vi "LEP_RV_CGen.vi"(7 "Rebuild":bool, 8 "error in (no error)":errorcluster, 9 "Top Level VI":path, 10 "Destination Folder":path, 11 "Configuration":T2={"Enable debugging"=FALSE, "Debug Options"=0, "Use stack variables"=FALSE, "Generate serial only"=FALSE, "Generate guard code"=TRUE, "Generate Integer Only"=TRUE, "Generate C Function Calls"=TRUE, "ExpressionFolding"=FALSE, "Constant Allocation"=0, "Constant Deallocation"=0, "Build Specification ID"="", "Preprocessor symbols (define)"="", "Compiler Flags"="", "Linker Flags"="", "Mode"=1, "Optimization"=2, "Optimize for time"=FALSE, "Enable cross-module optimization"=FALSE, "Include paths"=[], "Optimize heap size"=TRUE, "Use MicroLib"=FALSE, "Debug Mode"=2, "Enable profile information"=FALSE, "Host name"="board", "Use DHCP"=TRUE, "IP address"="0.0.0.0", "Subnet mask"="", "Gateway"="0.0.0.0", "Primary DNS"="0.0.0.0", "Secondary DNS"="0.0.0.0", "MAC in target memory"=TRUE, "MAC address"="", "Console output"=1, "Target serial port"=1} {"Constant Deallocation" items=["Out of Scope", "VI End", "Application End"]; "Constant Allocation" items=["First Use", "Containing Loop", "VI Initialization", "Application Initialization"]; "Target serial port" items=["0", "1", "2", "3"]; "Console output" items=["Processor status window", "Serial port"]; "Optimization" items=["Level 0 (-O0)", "Level 1 (-O1)", "Level 2 (-O2)", "Level 3 (-O3)"]; "Mode" items=["ARM-Mode", "Thumb-Mode"]; "Debug Options" items=["Use ULINK Debugger", "Use Simulator"]; "Debug Mode" items=["Instrumented (serial port)", "Instrumented (TCP/IP)", "Non-instrumented (JTAG/USB)"]}) -> (0 "error out":errorcluster, 1 "Error Indicator":bool[](array[boolean]), 2 "Status":T3(ring)=enum."EmptyTopLevelVIPath", 3 "Configuration":T2={"Enable debugging"=FALSE, "Debug Options"=0, "Use stack variables"=FALSE, "Generate serial only"=FALSE, "Generate guard code"=TRUE, "Generate Integer Only"=TRUE, "Generate C Function Calls"=TRUE, "ExpressionFolding"=FALSE, "Constant Allocation"=0, "Constant Deallocation"=0, "Build Specification ID"="", "Preprocessor symbols (define)"="", "Compiler Flags"="", "Linker Flags"="", "Mode"=1, "Optimization"=2, "Optimize for time"=FALSE, "Enable cross-module optimization"=FALSE, "Include paths"=[], "Optimize heap size"=TRUE, "Use MicroLib"=FALSE, "Debug Mode"=2, "Enable profile information"=FALSE, "Host name"="board", "Use DHCP"=TRUE, "IP address"="0.0.0.0", "Subnet mask"="", "Gateway"="0.0.0.0", "Primary DNS"="0.0.0.0", "Secondary DNS"="0.0.0.0", "MAC in target memory"=TRUE, "MAC address"="", "Console output"=1, "Target serial port"=1} {"Constant Deallocation" items=["Out of Scope", "VI End", "Application End"]; "Constant Allocation" items=["First Use", "Containing Loop", "VI Initialization", "Application Initialization"]; "Target serial port" items=["0", "1", "2", "3"]; "Console output" items=["Processor status window", "Serial port"]; "Optimization" items=["Level 0 (-O0)", "Level 1 (-O1)", "Level 2 (-O2)", "Level 3 (-O3)"]; "Mode" items=["ARM-Mode", "Thumb-Mode"]; "Debug Options" items=["Use ULINK Debugger", "Use Simulator"]; "Debug Mode" items=["Instrumented (serial port)", "Instrumented (TCP/IP)", "Non-instrumented (JTAG/USB)"]}, 4 "Node ID List":i32[](array[numeric]), 5 "Message List":string[][](array[string]))   [LabVIEW 2011]
doc: "Invokes the LabVIEW C Code Generator. This VI is a wrapper VI for the GenerateCCodeVariant VI server call."
uses:
  LEP_RV_Config.ctl
  LEP_RV_CGen.ctl
  <vilib>/LabVIEW Targets/Embedded/Debug/DD/utils/EMB_Debug_DD_GetSetAttrib_Numeric.vi
panel:
  in  "Config":T1={"TargetName"="", "GenerateDebugInfo"=FALSE, "GenerateGuardCode"=FALSE, "GenerateSerialOnly"=FALSE, "UseStackVariables"=FALSE, "MemoryModel"=0, "DestinationFolder"=path "", "GenerateIntegerOnly"=FALSE, "interruptServiceRoutineVIs"=[], "GenerateInlinePrintf"=FALSE, "BigEndian"=FALSE, "GenerateCFunctionCalls"=FALSE, "IncrementalBuild"=FALSE, "OCDIComments"=FALSE, "TargetAlignment"=8, "dynamicVIs"=[], "ExpressionFolding"=FALSE, "ProfileEnable"=FALSE, "Optimize subVI calls"=FALSE, "ConstantAllocation"=0, "ConstantDeallocation"=0, "VariableManagerIP"="", "BuildSpecID"="", "Silent"=TRUE} {"ConstantDeallocation" items=["Out of Scope", "VI End", "Application End"]; "ConstantAllocation" items=["First Use", "Containing Loop", "VI Initialization", "Application Initialization"]}
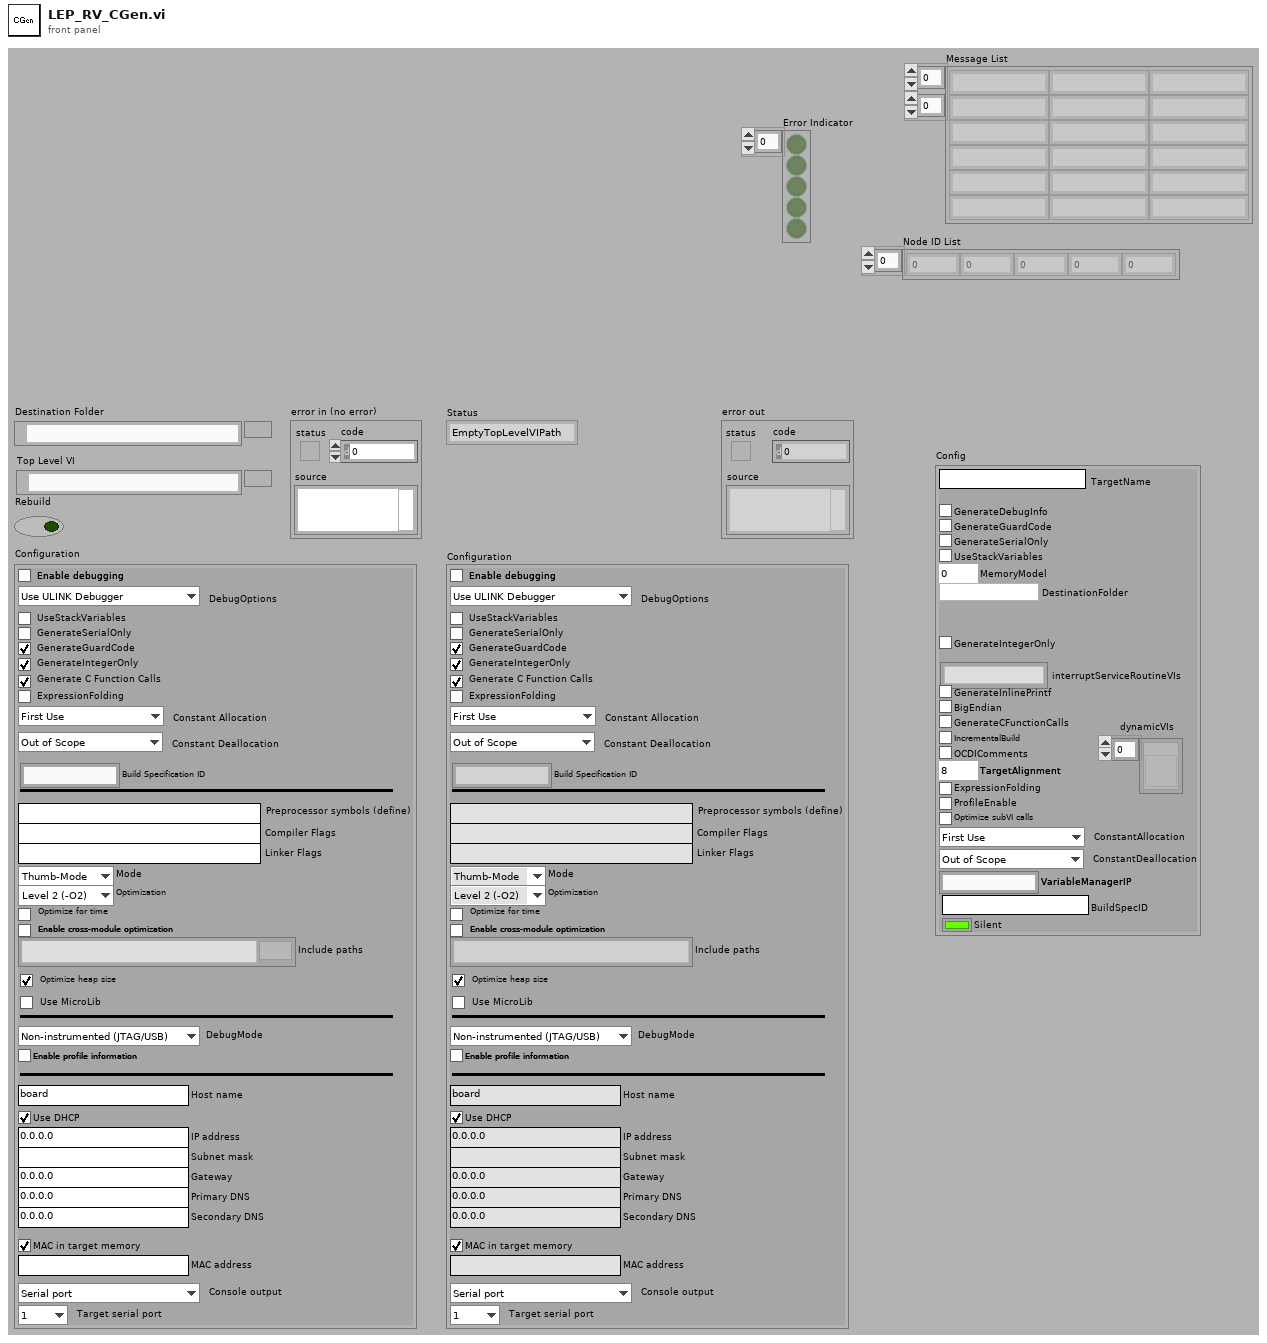
[diagram p1: front panel]
types:
  T1 = typedef "LEP_RV_CGen.ctl" = cluster{"TargetName":string, "GenerateDebugInfo":bool, "GenerateGuardCode":bool, "GenerateSerialOnly":bool, "UseStackVariables":bool, "MemoryModel":i32, "DestinationFolder":path, "GenerateIntegerOnly":bool, "interruptServiceRoutineVIs":path[], "GenerateInlinePrintf":bool, "BigEndian":bool, "GenerateCFunctionCalls":bool, "IncrementalBuild":bool, "OCDIComments":bool, "TargetAlignment":i32, "dynamicVIs":refnum<vi>[], "ExpressionFolding":bool, "ProfileEnable":bool, "Optimize subVI calls":bool, "ConstantAllocation":u16, "ConstantDeallocation":u16, "VariableManagerIP":string, "BuildSpecID":string, "Silent":bool}
  T2 = typedef "LEP_RV_Config.ctl" = cluster{"Enable debugging":bool, "Debug Options":u16, "Use stack variables":bool, "Generate serial only":bool, "Generate guard code":bool, "Generate Integer Only":bool, "Generate C Function Calls":bool, "ExpressionFolding":bool, "Constant Allocation":u16, "Constant Deallocation":u16, "Build Specification ID":string, "Preprocessor symbols (define)":string, "Compiler Flags":string, "Linker Flags":string, "Mode":u16, "Optimization":u16, "Optimize for time":bool, "Enable cross-module optimization":bool, "Include paths":path[], "Optimize heap size":bool, "Use MicroLib":bool, "Debug Mode":u16, "Enable profile information":bool, "Host name":string, "Use DHCP":bool, "IP address":string, "Subnet mask":string, "Gateway":string, "Primary DNS":string, "Secondary DNS":string, "MAC in target memory":bool, "MAC address":string, "Console output":u16, "Target serial port":u16}
  T3 = enum16{"NoErr", "TopLevelVIErr", "EmptyTopLevelVIPath", "CGenErr", "CpySuppFilesErr", "ProjectInfoErr", "NoTopLevelVIErr", "CreateBuildFolderErr", "EmptyBuildFolderErr", "LoadConfigErr", "BildToolsErr", "CompileErr", "LinkError", "DebugInfoErr", "NotFoundErr", "AccessErr", "ExecErr", "UnknownErr", "ISRErr"}
  T4 = enum16{"NoErr", "TopLevelVIErr", "EmptyTopLevelVIPath", "CGenErr", "CpySuppFilesErr", "ProjectInfoErr", "NoTopLevelVIErr", "CreateBuildFolderErr", "EmptyBuildFolderErr", "LoadConfigErr", "BildToolsErr", "CompileErr", "LinkError", "DebugInfoErr", "NotFoundErr", "AccessErr", "ExecErr", "UnknownErr"}
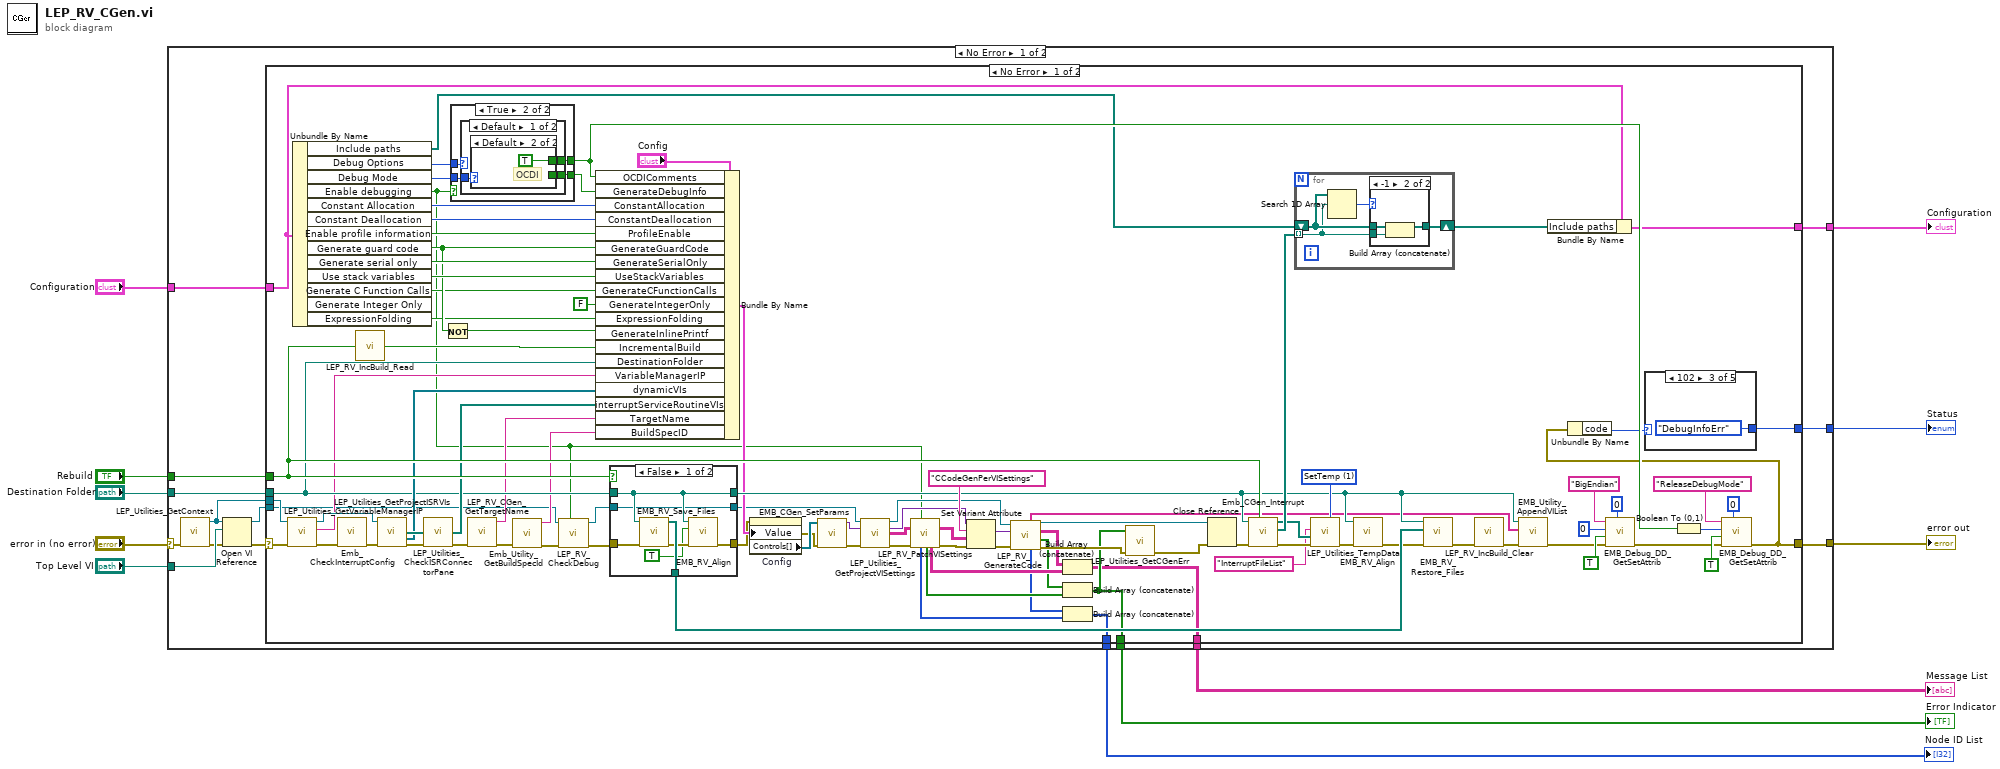
[diagram p0: block diagram]
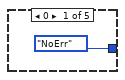
[diagram p2: hidden frame]
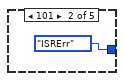
[diagram p3: hidden frame]
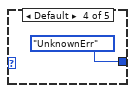
[diagram p4: hidden frame]
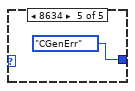
[diagram p5: hidden frame]
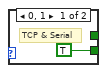
[diagram p7: hidden frame]
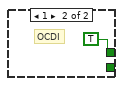
[diagram p8: hidden frame]
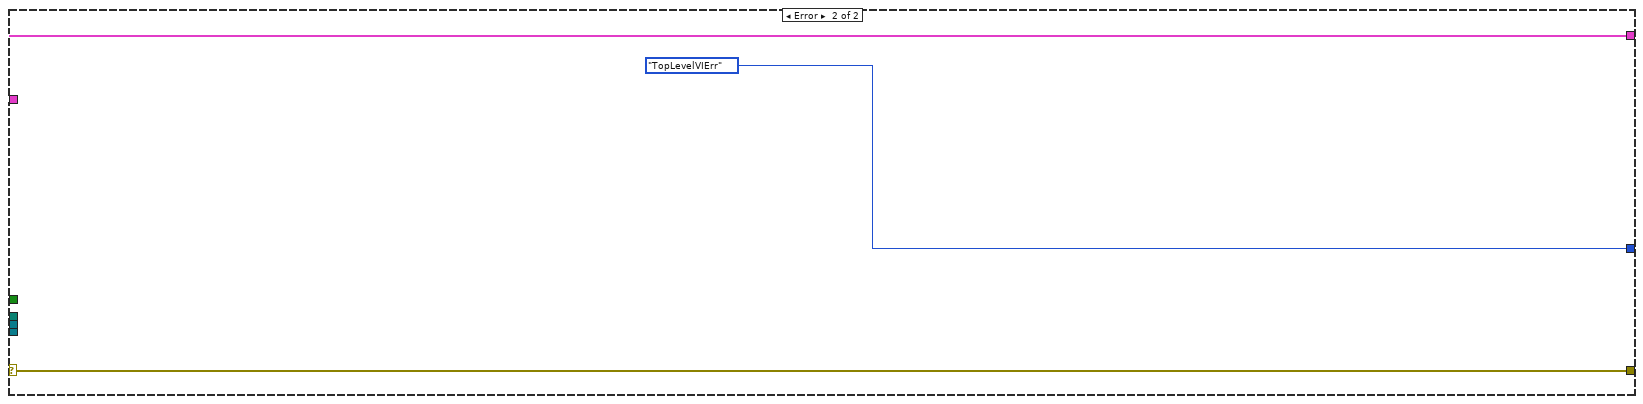
[diagram p11: hidden frame]
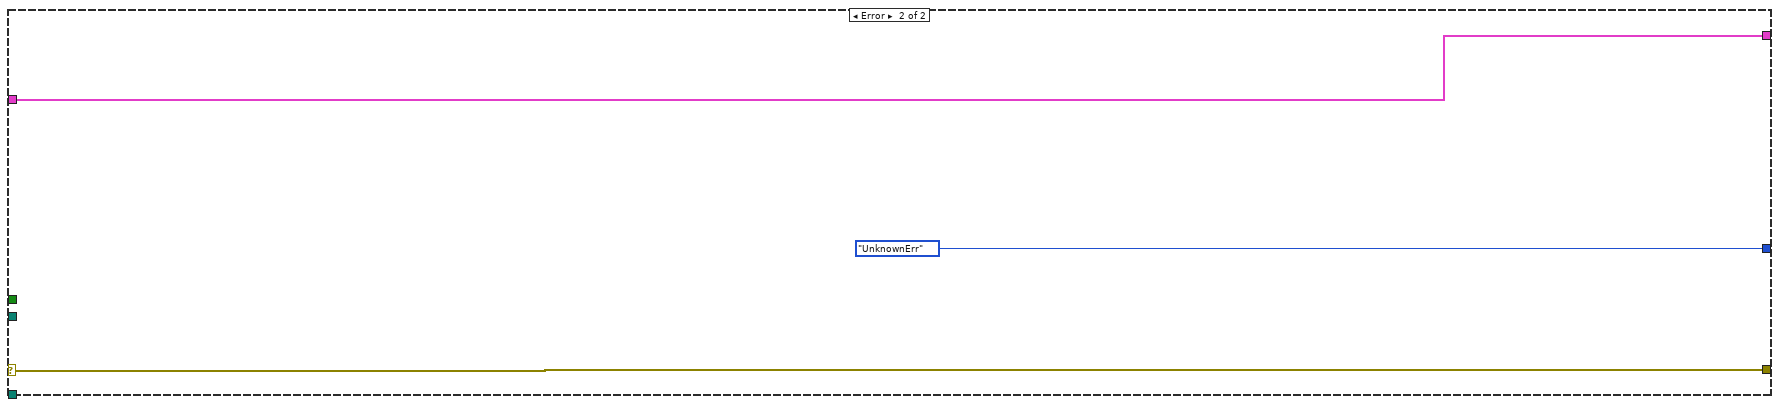
[diagram p12: hidden frame]
diagram:
  n1 = case shown="No Error" "error in (no error)" {
    selector: "error in (no error)" -> [w14 w160]
    tunnel: [w13 w160] -> w7
    tunnel: "Top Level VI" -> [w26 _]
    tunnel: "Destination Folder" -> [w24 _]
    tunnel: "Configuration" -> [w15 w158]
    tunnel: [w22 T4."UnknownErr" ("Errors")] -> w6
    tunnel: [w21 w158] -> w5
    tunnel: "Rebuild" -> [w19 _]
    tunnel: [w18 _] -> w1
    tunnel: [w17 _] -> w3
    tunnel: [w16 _] -> w2
    frame No Error {
      n2 = call <vilib>:"LEP_Utilities_GetContext.vi"("error in"=w14) -> ("error out"=w12:errorcluster, "Context"=w20:refnum<vi>)  [unwired: 9 out]
      n3 = Open VI Reference(application reference (local)=w20, vi path=w26, error in (no error)=w12) -> (vi reference=w25:refnum<vi>, error out=w23:errorcluster)  [unwired: 3 out]
      n4 = case shown="No Error" w23 {
        selector: w23 -> [w73 w157]
        tunnel: w25 -> [w42 _]
        tunnel: w24 -> [w76 _]
        tunnel: w15 -> [w102 w155]
        tunnel: [w46 w157] -> w13
        tunnel: [w60 T4."TopLevelVIErr" ("Errors")] -> w22
        tunnel: [w100 w155] -> w21
        tunnel: w20 -> [w72 _]
        tunnel: w19 -> [w87 _]
        tunnel: [w31 _] -> w18
        tunnel: [w27 _] -> w17
        tunnel: [w29 _] -> w16
        frame No Error {
          w98 = u16 1 items=["GetTemp", "SetTemp", "ClearTemp"] ("Command")
          n5 = call <vilib>:"LEP_Utilities_GetVariableManagerIP.vi"("error in (no error)"=w73, "application reference"=w72) -> ("error out"=w69:errorcluster, "address"=w70:string, "application reference out"=w71:refnum<vi>)  [unwired: 7 out]
          n6 = Unbundle By Name(w102) -> ("Include paths"=w104:path[], "Debug Options"=w85:u16, "Debug Mode"=w119:u16, "Enable debugging"=w36:bool, "Constant Allocation"=w75:u16, "Constant Deallocation"=w74:u16, "Enable profile information"=w77:bool, "Generate guard code"=w114:bool, "Generate serial only"=w117:bool, "Use stack variables"=w116:bool, "Generate C Function Calls"=w80:bool, "ExpressionFolding"=w79:bool)  [unwired: 1 out]
          n7 = call "Emb_CheckInterruptConfig.vi"("error in (no error)"=w69) -> ("error out"=w68:errorcluster)  [unwired: 10 out]
          n8 = call "LEP_RV_IncBuild_Read.vi"("Rebuild?"=w87) -> ("Incremental Build?"=w88:bool)
          n9 = call <vilib>:"LEP_Utilities_GetProjectISRVIs.vi"("Context"=w71, "error in"=w68) -> ("ISRFiles"=w120:path[], "Dynamic Files"=w86:refnum<vi>[], "error out"=w121:errorcluster)  [unwired: 11 out]
          n10 = call <vilib>:"LEP_Utilities_CheckISRConnectorPane.vi"("ISR VIs"=w120, "error in (no error)"=w121) -> ("ISR VIs Out"=w78:path[], "error out"=w63:errorcluster)  [unwired: 12 out]
          n11 = Not(x=w114) -> (.not. x?=w115:bool)
          n12 = case shown="True" w36 {
            tunnel: w119 -> [_ w130]
            tunnel: [_ w129] -> w118
            tunnel: [_ w128] -> w105
            tunnel: w85 -> [_ w127]
            frame False {
            }
            frame True {
              n13 = case shown="Default" w127 {
                tunnel: w130 -> [w133 _]
                tunnel: [w132 _] -> w129
                tunnel: [w131 TRUE] -> w128
                frame Default {
                  n14 = case shown="Default" w133 {
                    tunnel: [_ TRUE] -> w131
                    tunnel: [TRUE _] -> w132
                    frame 0, 1 {
                      # "TCP & Serial"
                    }
                    frame Default {
                      # "OCDI"
                    }
                  }
                }
                frame 1 {
                  # "OCDI"
                }
              }
            }
          }
          n15 = call "LEP_RV_CGen_GetTargetName.vi"("error in (no error)"=w63) -> ("error out"=w59:errorcluster, "App.TargetInfo"=w64:string)  [unwired: 2 in, 7 out]
          n16 = call <vilib>:"Emb_Utility_GetBuildSpecId.vi"("error in (no error)"=w59) -> ("error out"=w44:errorcluster, "buildSpec ID"=w58:string)  [unwired: 7 out]
          n17 = call "LEP_RV_CheckDebug.vi"("Enable debugging"=w36, "error in (no error)"=w44, "VI Refnum"=w42) -> ("error out"=w43:errorcluster, "VI Refnum out"=w41:refnum<vi>)  [unwired: 7 in]
          n18 = Bundle By Name(cluster="Config", "OCDIComments"=w105, "GenerateDebugInfo"=w118, "ConstantAllocation"=w75, "ConstantDeallocation"=w74, "ProfileEnable"=w77, "GenerateGuardCode"=w114, "GenerateSerialOnly"=w117, "UseStackVariables"=w116, "GenerateCFunctionCalls"=w80, "GenerateIntegerOnly"=FALSE, "ExpressionFolding"=w79, "GenerateInlinePrintf"=w115, "IncrementalBuild"=w88, "DestinationFolder"=w76, "VariableManagerIP"=w70, "dynamicVIs"=w86, "interruptServiceRoutineVIs"=w78, "TargetName"=w64, "BuildSpecID"=w58) -> (w51:T1)
          n19 = case shown="False" w87 {
            tunnel: w43 -> [w143 w144]
            tunnel: [w142 _] -> w99
            tunnel: [w140 w144] -> w48
            tunnel: w76 -> [w138 w146]
            tunnel: [w138 w146] -> w67
            tunnel: w41 -> [w137 w145]
            tunnel: [w137 w145] -> w47
            frame False {
              n20 = call <vilib>:"EMB_RV_Save_Files.vi"("error in (no error)"=w143, "destination folder"=w138) -> ("error out"=w141:errorcluster, "temporary paths"=w142:path[])  [unwired: 8 out]
              n21 = call <vilib>:"EMB_RV_Align.vi"("error in (no error)"=w141, "undo alignment"=TRUE, "Path"=w138) -> ("error out"=w140:errorcluster)  [unwired: 8 out]
            }
            frame True {
            }
          }
          n22 = property on="Config" class="Clust (strict)"(error in=w48, "Value"=w51) -> (error out=w49:errorcluster, "Controls[]"=w50:refnum<vi>[])  [unwired: 1 in, 1 out]
          n23 = call <vilib>:"EMB_CGen_SetParams.vi"("error in (no error)"=w49, "Controls[]"=w50) -> ("error out"=w93:errorcluster, "Config out"=w84:variant)  [unwired: 8 out]
          n24 = call <vilib>:"LEP_Utilities_GetProjectVISettings.vi"("Top Level VI"=w47, "Config In"=w84, "error in"=w93) -> ("Cloned Top Level VI"=w82:refnum<vi>, "Config Out"=w83:variant, "CGen Info Array"=w38:string[][], "error out"=w40:errorcluster)  [unwired: 2 in, 7 out]
          n25 = call "LEP_RV_PatchVISettings.vi"("Enable debugging"=w36, "CGen Info Array"=w38, "error in (no error)"=w40) -> ("CGen Info Array out"=w37:string[][], "Node ID List"=w35:i32[], "Error Indicator"=w34:bool[], "Message List"=w33:string[][], "error out"=w39:errorcluster)  [unwired: 8 in]
          n26 = Set Variant Attribute(Variant=w83, name="CCodeGenPerVISettings", value=w37, error in=w39) -> (Variant out=w92:variant, error out=w57:errorcluster)  [unwired: 1 out]
          n27 = call "LEP_RV_GenerateCode.vi"("error out 2"=w57, "Config Out"=w92, "Cloned Top Level VI 2"=w82) -> ("error out"=w56:errorcluster, "Warning List"=w30:bool[], "Error List"=w28:string[][], "Cloned Top Level VI"=w54:refnum<vi>, "Node ID List"=w32:i32[], "fileList"=w53:string[])  [unwired: 3 in]
          n28 = Build Array (concatenate)(w28, w33) -> (w27:string[][])
          n29 = Build Array (concatenate)(w30, w34) -> (w29:bool[])
          n30 = Build Array (concatenate)(w32, w35) -> (w31:i32[])
          n31 = call <vilib>:"LEP_Utilities_GetCGenErr.vi"("error in"=w56, "Error Indicator"=w29) -> ("error out"=w55:errorcluster)  [unwired: 9 in]
          n32 = Close Reference(reference=w54, error in (no error)=w55) -> (error out=w91:errorcluster)
          n33 = call "Emb_CGen_Interrupt.vi"("Rebuild"=w87, "error in (no error)"=w91, "Destination Directory"=w67) -> ("error out"=w97:errorcluster, "include folders"=w103:path[], "source files"=w96:path[])  [unwired: 6 out]
          n34 = for {
            shift-right: [w147] -> w101
            shift-left: w104 -> [w149]
            tunnel: w103 -> [w148] mode=indexing
            n35 = Search 1D Array(1D array=w149, element=w148) -> (index of element=w150:i32)  [unwired: 1 out]
            n36 = case shown="-1" w150 {
              tunnel: w149 -> [w151 w153]
              tunnel: w148 -> [_ w154]
              tunnel: [w151 w152] -> w147
              frame 0, Default {
              }
              frame -1 {
                n37 = Build Array (concatenate)(w153, w154) -> (w152:path[])
              }
            }
          }
          n38 = call <vilib>:"LEP_Utilities_TempData.vi"("error in"=w97, "Variant In"=w96, "Name"="InterruptFileList", "Command"=w98) -> ("error out"=w90:errorcluster)  [unwired: 1 in, 6 out]
          n39 = call <vilib>:"EMB_RV_Align.vi"("error in (no error)"=w90, "Path"=w67) -> ("error out"=w89:errorcluster)  [unwired: 1 in, 8 out]
          n40 = call <vilib>:"EMB_RV_Restore_Files.vi"("error in (no error)"=w89, "temporary paths"=w99, "destination folder"=w67) -> ("error out"=w66:errorcluster)  [unwired: 8 out]
          n41 = call "LEP_RV_IncBuild_Clear.vi"("error in (no error)"=w66) -> ("error out"=w65:errorcluster)  [unwired: 10 out]
          n42 = call <vilib>:"EMB_Utility_AppendVIList.vi"("error in (no error)"=w65, "VI List"=w53, "Build Path"=w67) -> ("error out"=w62:errorcluster)  [unwired: 8 out]
          n43 = Bundle By Name(cluster=w102, "Include paths"=w101) -> (w100:T2)
          n44 = call-poly <vilib>:"EMB_Debug_DD_GetSetAttrib.vi"("target ID"=u32 0, "error in (no error)"=w62, "set"=TRUE, "value"=0, "name"="BigEndian") -> ("error out"=w106:errorcluster)  [unwired: 6 out]
          n45 = Boolean To (0,1)(Boolean=w105) -> (0, 1=w111:i16)
          n46 = call-poly <vilib>:"EMB_Debug_DD_GetSetAttrib.vi"("target ID"=u32 0, "error in (no error)"=w106, "set"=TRUE, "value"=w111, "name"="ReleaseDebugMode") -> ("error out"=w46:errorcluster)  [unwired: 6 out]
          n47 = Unbundle By Name(w46) -> ("code"=w61:i32)
          n48 = case shown="102" w61 {
            tunnel: [T3."NoErr" ("Errors") T3."ISRErr" ("Errors") T3."DebugInfoErr" ("Errors") T3."UnknownErr" ("Errors") T3."CGenErr" ("Errors")] -> w60
            frame 0 {
            }
            frame 101 {
            }
            frame 102 {
            }
            frame Default {
            }
            frame 8634 {
            }
          }
        }
        frame Error {
        }
      }
    }
    frame Error {
    }
  }
  "error out" <- w7
  "Status" <- w6
  "Configuration" <- w5
  "Node ID List" <- w1
  "Error Indicator" <- w2
  "Message List" <- w3
